vi "get_ref.vi"(11 "Item in":refnum<class "Item.lvclass">) -> (2 "ref":u64)   [LabVIEW 2020, in "toml_edit.lvlib" / "Item.lvclass"]
uses:
  Item.lvclass
  Item.lvclass/Item.ctl
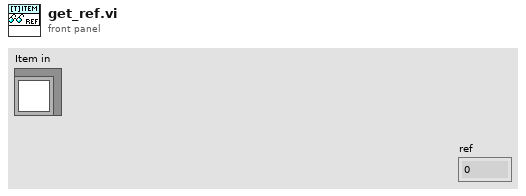
[diagram p1: front panel]
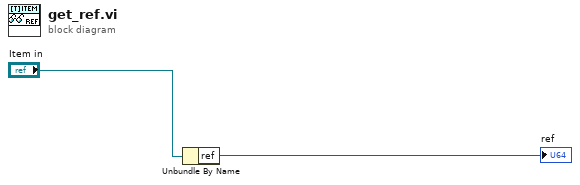
[diagram p0: block diagram]
diagram:
  n1 = Unbundle By Name("Item in") -> ("ref"=→"ref":u64)
